vi "Delete Uint16 DVR.vi"(8 "error in (no error)":errorcluster, 11 "Uint16 DVR in":refnum<data-value>) -> (0 "error out":errorcluster, 3 "Uint16 out":refnum<class "Uint16.lvclass">)   [LabVIEW 2015, in "MDSplus.lvlib" / "Uint16.lvclass"]
uses:
  Uint16.lvclass
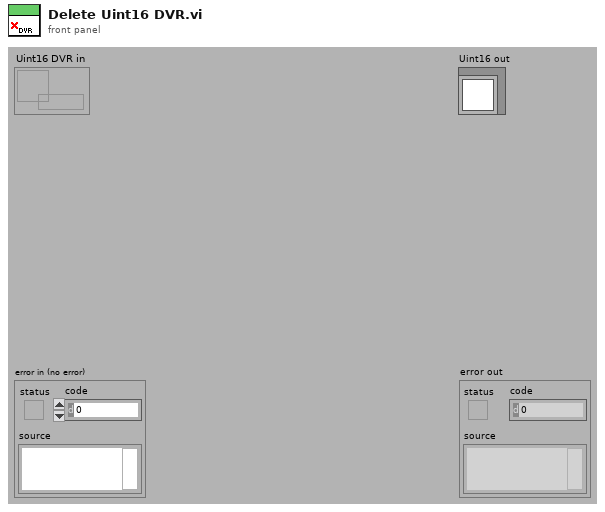
[diagram p1: front panel]
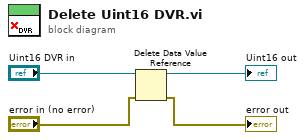
[diagram p0: block diagram]
diagram:
  n1 = Delete Data Value Reference(data value reference="Uint16 DVR in", error in="error in (no error)") -> (data value=→"Uint16 out":refnum<class "Uint16.lvclass">, error out=→"error out":errorcluster)
